vi "Complete Multipart Upload.vi"(8 "error in (no error)":errorcluster, 11 "Multipart Upload RefNum in":T2) -> (0 "error out":errorcluster, 1 "Version ID":string, 2 "CompleteMultipartUploadResult":T1, 3 "Multipart Upload RefNum out":T2)   [LabVIEW 2011, in "LV Interface for Amazon S3.lvlib"]
doc: "This operation completes a multipart upload by assembling previously uploaded parts. <B>You must initiate a multipart upload</B> (see Initiate Multipart Upload.vi) <B> and upload all parts before you complete a multipart upload</B>. <B>After</B> that, you have to <B>free up resources</B> on your system <B>by closing the multipart upload reference</B> (see Close Multipart Upload Reference.vi)"
uses:
  LV Interface for Amazon S3.lvlib
  Typedefs/AMZ_S3_Multipart Upload RefNum.ctl
  Typedefs/AMZ_S3_Multipart Upload RefNum Enum.ctl
  Typedefs/AMZ_S3_API_CompleteMultipartUploadResult.ctl
  Typedefs/AMZ_S3_HTTP Header-Value pair.ctl
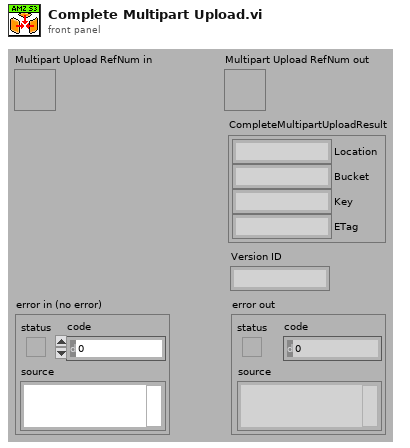
[diagram p1: front panel]
types:
  T1 = typedef "LV Interface for Amazon S3.lvlib/AMZ_S3_API_CompleteMultipartUploadResult.ctl" = cluster{"Location":string, "Bucket":string, "Key":string, "ETag":string}
  T2 = typedef "LV Interface for Amazon S3.lvlib/AMZ_S3_Multipart Upload RefNum.ctl" = refnum<k1>
  T3 = typedef "LV Interface for Amazon S3.lvlib/AMZ_S3_HTTP Header-Value pair.ctl" = cluster{"Header":string, "Value":string}
  T4 = typedef "LV Interface for Amazon S3.lvlib/AMZ_S3_Multipart Upload Data.ctl" = cluster{"Object":string, "Bucket":string, "UploadID":string, "Parts":T5[]}
  T5 = typedef "LV Interface for Amazon S3.lvlib/AMZ_S3_Multipart Upload Part Data.ctl" = cluster{"PartNumber":u16, "Lat modified":timestamp, "ETag":string, "Size":u64}
  T6 = typedef "LV Interface for Amazon S3.lvlib/AMZ_S3_Call Results.ctl" = enum16{"Success", "UndefinedError", "AccessDenied", "AccountProblem", "AmbiguousGrantByEmailAddress", "BadDigest", "BucketAlreadyExists", "BucketAlreadyOwnedByYou", "BucketNotEmpty", "CredentialsNotSupported", "CrossLocationLoggingProhibited", "EntityTooSmall", "EntityTooLarge", "ExpiredToken", "IllegalVersioningConfigurationException", "IncompleteBody", "IncorrectNumberOfFilesInPostRequest", "InlineDataTooLarge", "InternalError", "InvalidAccessKeyId", "InvalidAddressingHeader", "InvalidArgument", "InvalidBucketName", "InvalidDigest", "InvalidLocationConstraint", "InvalidPart", "InvalidPartOrder", "InvalidPayer", "InvalidPolicyDocument", "InvalidRange", "InvalidSecurity", "InvalidSOAPRequest", "InvalidStorageClass", "InvalidTargetBucketForLogging", "InvalidToken", "InvalidURI", "KeyTooLong", "MalformedACLError", "MalformedPOSTRequest", "MalformedXML", "MaxMessageLengthExceeded", "MaxPostPreDataLengthExceededError", "MetadataTooLarge", "MethodNotAllowed", "MissingAttachment", "MissingContentLength", "MissingRequestBodyError", "MissingSecurityElement", "MissingSecurityHeader", "NoLoggingStatusForKey", "NoSuchBucket", "NoSuchKey", "NoSuchUpload", "NoSuchVersion", "NotImplemented", "NotSignedUp", "OperationAborted", "PermanentRedirect", "PreconditionFailed", "Redirect", "RequestIsNotMultiPartContent", "RequestTimeout", "RequestTimeTooSkewed", "RequestTorrentOfBucketError", "SignatureDoesNotMatch", "SlowDown", "TemporaryRedirect", "TokenRefreshRequired", "TooManyBuckets", "UnexpectedContent", "UnresolvableGrantByEmailAddress", "UserKeyMustBeSpecified", "LabVIEWError"}
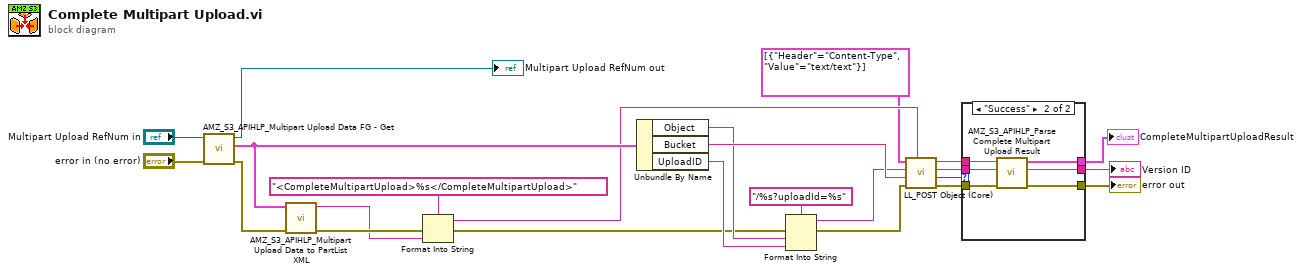
[diagram p0: block diagram]
diagram:
  n1 = call "AMZ_S3_APIHLP_Multipart Upload Data FG - Get.vi"("error in (no error)"="error in (no error)", "Multipart Upload RefNum in"="Multipart Upload RefNum in") -> ("error out"=w16:errorcluster, "Multipart Upload Data"=w15:T4, "Multipart Upload RefNum out"=→"Multipart Upload RefNum out":T2)  [unwired: 7 in]
  n2 = call "AMZ_S3_APIHLP_Multipart Upload Data to PartList XML.vi"("error in (no error)"=w16, "Multipart Upload Data"=w15) -> ("error out"=w13:errorcluster, "PartList XML"=w12:string)  [unwired: 8 in]
  n3 = Format Into String(format string="<CompleteMultipartUpload>%s</CompleteMultipartUpload>", error in=w13, w12) -> (resulting string=w10:string, error out=w11:errorcluster)  [unwired: 1 in]
  n4 = Unbundle By Name(w15) -> ("Object"=w19:string, "Bucket"=w22:string, "UploadID"=w20:string)
  n5 = Format Into String(format string="/%s?uploadId=%s", error in=w11, w19, w20) -> (resulting string=w17:string, error out=w18:errorcluster)  [unwired: 1 in]
  n6 = call "LL_POST Object (Core).vi"("Data"=w10, "error in (no error)"=w18, "Bucket"=w22, "Path"=w17, "Headers"=T3[] [{"Header"="Content-Type", "Value"="text/text"}]) -> ("error out"=w7:errorcluster, "Call Result"=w8:T6, "Response body"=w5:string, "Response header"=w6:string)  [unwired: 3 in]
  n7 = case shown="\"Success\"" w8 {
    tunnel: w7 -> [w25 w30]
    tunnel: w6 -> [_ w31]
    tunnel: w5 -> [_ w29]
    tunnel: [_ w28] -> w3
    tunnel: [w25 w27] -> w4
    tunnel: [_ w26] -> w1
    frame Default {
    }
    frame "Success" {
      n8 = call "AMZ_S3_APIHLP_Parse Complete Multipart Upload Result.vi"("error in (no error)"=w30, "Response body"=w29, "Response header"=w31) -> ("error out"=w27:errorcluster, "Version ID"=w26:string, "CompleteMultipartUploadResult"=w28:T1)  [unwired: 6 in]
    }
  }
  "error out" <- w4
  "CompleteMultipartUploadResult" <- w3
  "Version ID" <- w1
